vi "BRig_dataLC_Cue_First_Delay_l1.vi"() -> (2 "output_Cue_First_Delay":i32)   [LabVIEW 2014]
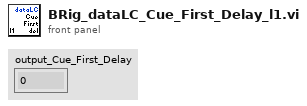
[diagram p1: front panel]
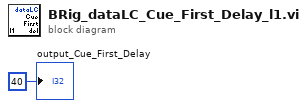
[diagram p0: block diagram]
diagram:
  "output_Cue_First_Delay" <- 40 ("output_iBlock")
